vi "GT Laser Power Mode.vi"(5 "delaymode":i16, 6 "channel":i16, 7 "minValue":dbl, 8 "error in (no error)":errorcluster caption="错误输入（无错误）", 9 "maxValue":dbl, 10 "laserPowerMode":i16, 11 "cardNum":i16) -> (0 "error out":errorcluster caption="错误输出", 3 "function return":i16)   [LabVIEW 2014, in "gts.lvlib"]
doc: "GT_API GT_LaserPowerMode(short cardNum,short laserPowerMode,double maxValue,double minValue,short channel=0,short delaymode =0);"
uses:
  gts.lvlib
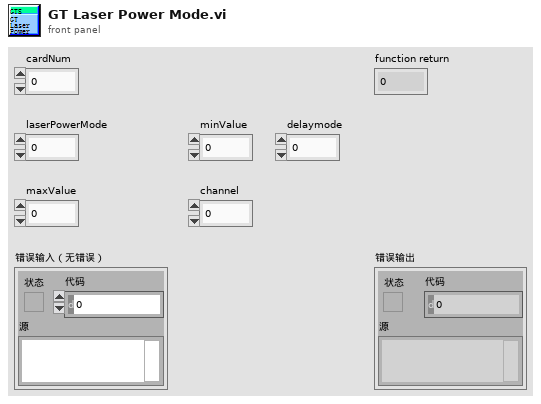
[diagram p1: front panel]
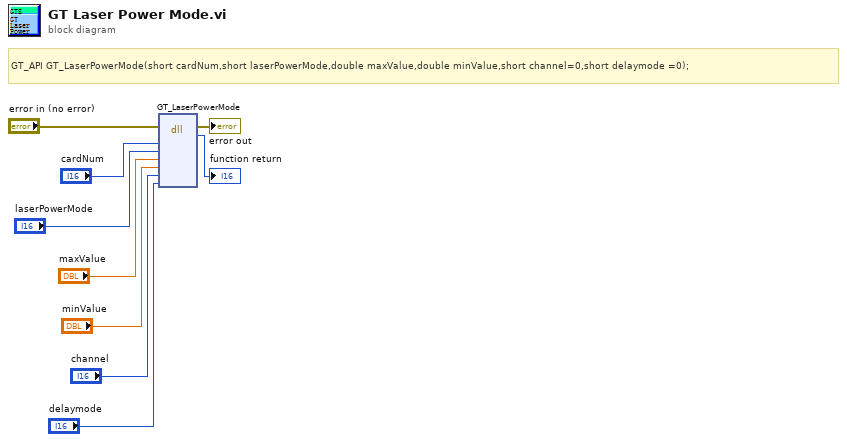
[diagram p0: block diagram]
diagram:
  # "GT_API GT_LaserPowerMode(short cardNum,short laserPowerMode,double maxValue,double minValue,short channel=0,short delaymode =0);"
  n1 = dll-call lib="PTH2habs D固高科技资料GTS控制卡GTS卡18年上半年资料dllVC32bit\nmulti_cardgts.*" fn="GT_LaserPowerMode"(error in="error in (no error)", "cardNum"="cardNum", "laserPowerMode"="laserPowerMode", "maxValue"="maxValue", "minValue"="minValue", "channel"="channel", "delaymode"="delaymode") -> (error out=→"error out":errorcluster, →"function return":i16)  [unwired: 8 in, 1 out]
